vi "Launch Analyze.vi"(7 "Chart Ref":refnum<vi>, 8 "error in (no error)":errorcluster) -> (0 "error out":errorcluster, 3 "appended path":path)   [LabVIEW 2014]
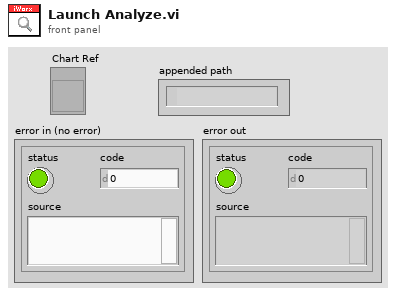
[diagram p1: front panel]
types:
  T1 = enum32{"Invalid", "Standard", "Closed", "Hidden", "Minimized", "Maximized"}
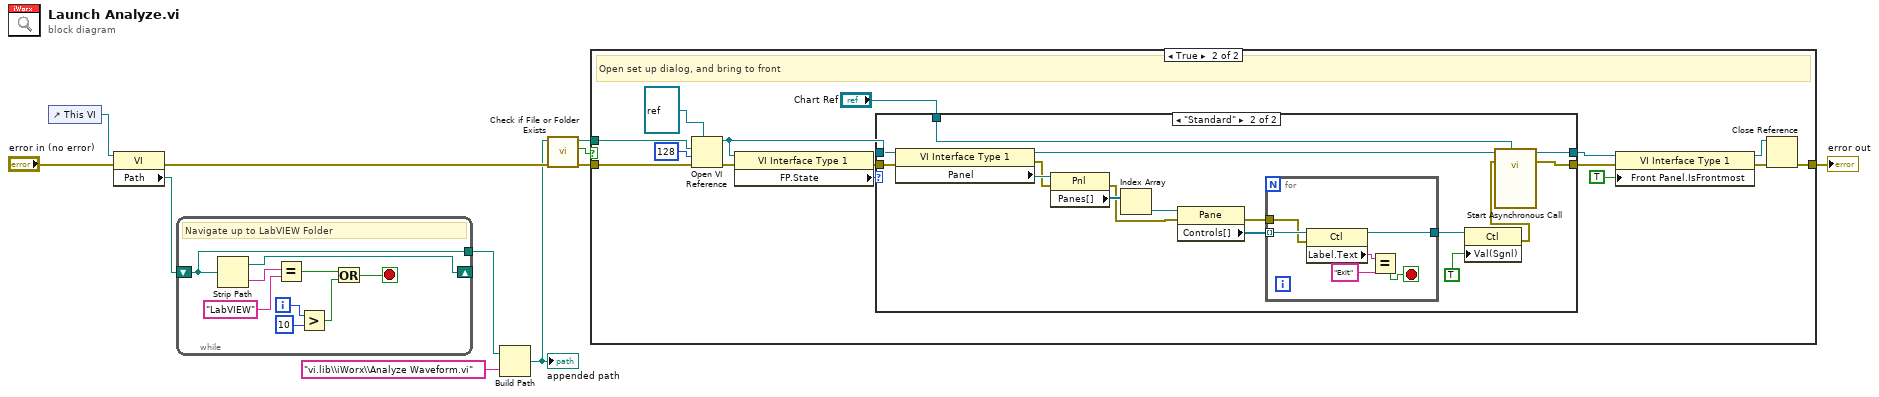
[diagram p0: block diagram]
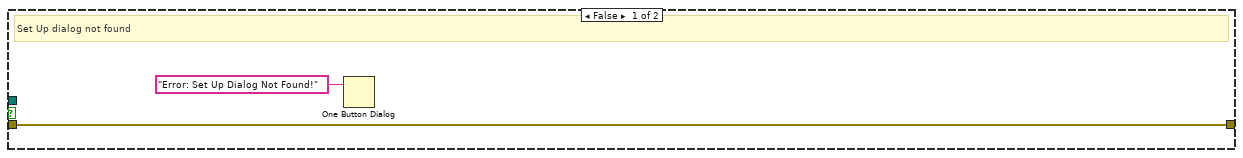
[diagram p2: hidden frame]
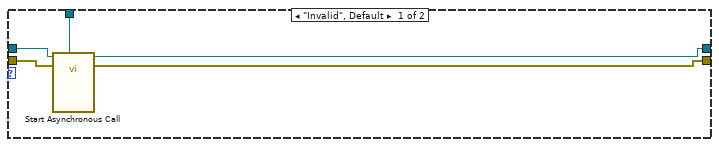
[diagram p3: hidden frame]
diagram:
  n1 = control-ref of="This VI"() -> (w8:refnum<vi>)
  n2 = property class="VI"(reference=w8, error in="error in (no error)") -> (error out=w5:errorcluster, "Path"=w9:path)  [unwired: 1 out]
  n3 = while {
    shift-right: [w20] -> _
    shift-left: w9 -> [w17]
    tunnel: [w17] -> w11
    i -> [w15]
    stop <- w12 stop-if-true
    # "Navigate up to LabVIEW Folder"
    n4 = Strip Path(path=w17) -> (stripped path=w20:path, name=w19:string)
    n5 = Equal?(x=w19, y="LabVIEW" ("name or relative path")) -> (x = y?=w16:bool)
    n6 = Greater?(x=w15, y=10) -> (0:w13:bool)
    n7 = Or(x=w16, y=w13) -> (x .or. y?=w12:bool)
  }
  n8 = Build Path(base path=w11, name or relative path="vi.lib\\iWorx\\Analyze Waveform.vi") -> (appended path=w1:path)
  "appended path" <- w1
  n9 = call <vilib>:"Check if File or Folder Exists.vi"("error in (no error)"=w5, "path"=w1) -> ("error out"=w3:errorcluster, "file or folder exists?"=w2:bool, "dup path"=w4:path)  [unwired: 7 in]
  n10 = case shown="True" w2 {
    tunnel: [w22 w36] -> w7
    tunnel: w4 -> [_ w34]
    tunnel: w3 -> [w22 w33]
    frame False {
      # "Set Up dialog not found"
      n11 = One Button Dialog(message="Error: Set Up Dialog Not Found!") -> ()  [unwired: 1 in, 1 out]
    }
    frame True {
      # "Open set up dialog, and bring to front"
      n12 = Open VI Reference(type specifier VI Refnum (for type only)=refnum<vi> refnum, vi path=w34, options=128, error in (no error)=w33) -> (vi reference=w27:refnum<vi>, error out=w25:errorcluster)  [unwired: 2 in]
      n13 = property class="VI Interface Type 1"(reference=w27, error in=w25) -> (error out=w24:errorcluster, "FP.State"=w26:T1)  [unwired: 1 out]
      n14 = case shown="\"Standard\"" w26 {
        tunnel: w24 -> [w42 w50]
        tunnel: [w41 w57] -> w32
        tunnel: [w40 w56] -> w30
        tunnel: w27 -> [w39 w55]
        tunnel: "Chart Ref" -> [w38 w58]
        frame "Invalid", Default {
          n15 = call-by-ref "Start Asynchronous Call"(reference=w39, error in=w42, "Chart Ref"=w38) -> (reference out=w41:refnum<vi>, error out=w40:errorcluster)  [unwired: 11 in]
        }
        frame "Standard" {
          n16 = property class="VI Interface Type 1"(reference=w55, error in=w50) -> (reference out=w51:refnum<vi>, error out=w49:errorcluster, "Panel"=w54:refnum<vi>)
          n17 = property class="Pnl"(reference=w54, error in=w49) -> (error out=w48:errorcluster, "Panes[]"=w53:refnum<vi>[])  [unwired: 1 out]
          n18 = Index Array(array=w53) -> (element=w52:refnum<vi>)  [unwired: 1 in]
          n19 = property class="Pane"(reference=w52, error in=w48) -> (error out=w46:errorcluster, "Controls[]"=w47:refnum<vi>[])  [unwired: 1 out]
          n20 = for {
            tunnel: w47 -> [w64] mode=indexing
            tunnel: w46 -> [w63]
            tunnel: [w59] -> w45
            stop <- w60 stop-if-true
            n21 = property class="Ctl"(reference=w64, error in=w63) -> (reference out=w59:refnum<vi>, "Label.Text"=w62:string)  [unwired: 1 out]
            n22 = Equal?(x=w62, y="Exit") -> (x = y?=w60:bool)
          }
          n23 = property class="Ctl"(reference=w45, "Val(Sgnl)"=TRUE) -> (error out=w43:errorcluster)  [unwired: 1 in, 1 out]
          n24 = call-by-ref "Start Asynchronous Call"(reference=w51, error in=w43, "Chart Ref"=w58) -> (reference out=w57:refnum<vi>, error out=w56:errorcluster)  [unwired: 11 in]
        }
      }
      n25 = property class="VI Interface Type 1"(reference=w32, error in=w30, "Front Panel.IsFrontmost"=TRUE ("Front Panel Window:Is Frontmost")) -> (reference out=w31:refnum<vi>, error out=w29:errorcluster)
      n26 = Close Reference(reference=w31, error in (no error)=w29) -> (error out=w36:errorcluster)
    }
  }
  "error out" <- w7
